vi "getFilePaths.vi"(8 "error in (no error)":errorcluster, 11 "reference in":refnum<class "File Controller.lvclass">) -> (0 "error out":errorcluster, 3 "reference out":refnum<class "File Controller.lvclass">)   [LabVIEW 2015, in "File Controller.lvclass"]
uses:
  File Controller.lvclass
  <vilib>/Utility/config.llb/Read Key (Path).vi
  <vilib>/Utility/config.llb/NI_LVConfig.lvlib
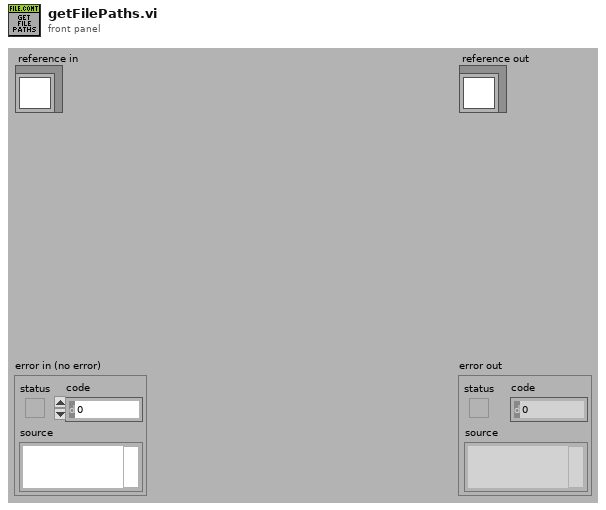
[diagram p1: front panel]
types:
  T1 = typedef "File Controller.lvclass/ObjectAttributesRef.ctl" = refnum<data-value>
  T2 = typedef "File Controller.lvclass/ObjectAttributes.ctl" = cluster{"MyAttribute":dbl, "excelFile_refs":refnum<class "excelFile.lvclass">[], "filePaths":path[], "outlookTemplatePaths":path[], "attachmentTemplatePaths":path[], "configFilePath":path, "not_setting":bool[], "python_ref":refnum<class "python.lvclass">, "TSR":cluster{"number":string, "TSR_path":path, "service_path":path, "email_to":string}}
  T3 = typedef "NI_LVConfig.lvlib/Config Data RefNum.ctl" = refnum<k1>
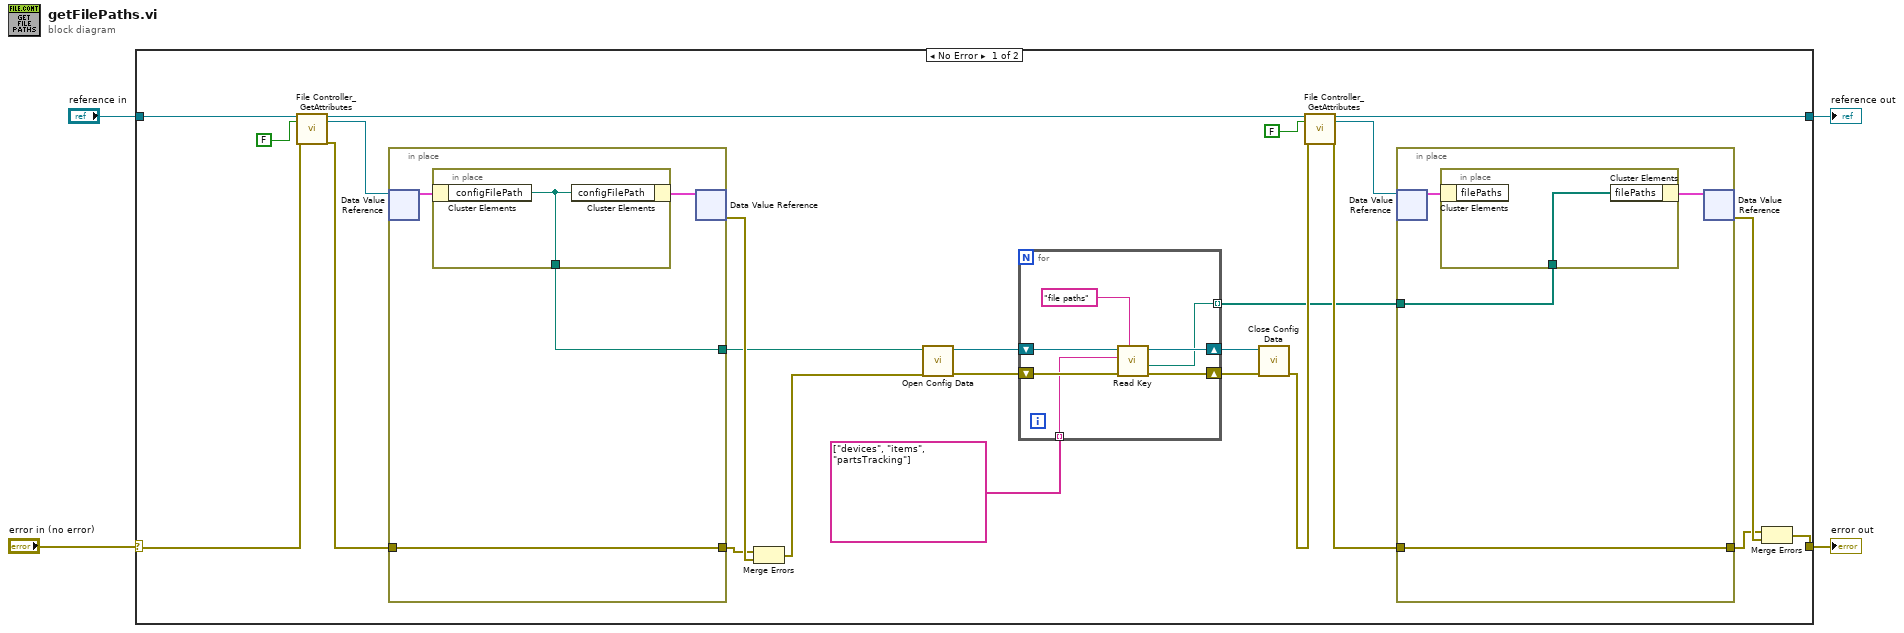
[diagram p0: block diagram]
diagram:
  n1 = case shown="No Error" "error in (no error)" {
    selector: "error in (no error)" -> [w9 w47]
    tunnel: [w28 w47] -> w3
    tunnel: [w23 w46] -> w1
    tunnel: "reference in" -> [w8 w46]
    frame No Error {
      n2 = call "File Controller_GetAttributes.vi"("reference in"=w8, "return data? (T)"=FALSE, "error in (no error)"=w9) -> ("reference out"=w7:refnum<class "File Controller.lvclass">, "attributes ref"=w10:T1, "error out"=w11:errorcluster)  [unwired: 13 in, 1 out]
      n3 = in-place {
        in-place-border: w11 -> [w30]
        in-place-border: [w30] -> w13
        in-place-border: [w29] -> w6
        n4 = in-place-dvr #1(w10) -> (w31:T2)  [unwired: 1 out]
        n5 = in-place {
          in-place-border: [w33] -> w29
          n6 = in-place-cluster #2(w31) -> ("configFilePath"=w33:path)
          n7 = in-place-cluster #2("configFilePath"=w33) -> (w32:T2)
        }
        n8 = in-place-dvr #1(w32) -> (w14:errorcluster)  [unwired: 1 out]
      }
      n9 = Merge Errors(w13, w14) -> (w5:errorcluster)
      n10 = call <vilib>:"Open Config Data.vi"("error in (no error)"=w5, "configuration file path"=w6) -> ("error out"=w20:errorcluster, "refnum"=w21:T3)  [unwired: 7 in, 1 out]
      n11 = for {
        shift-right: [w37] -> w19
        shift-left: w21 -> [w40]
        shift-right: [w36] -> w18
        shift-left: w20 -> [w39]
        tunnel: string[] ["devices", "items", "partsTracking"] -> [w35] mode=indexing
        tunnel: [w34] -> w15 mode=indexing
        n12 = call-poly <vilib>:"Read Key.vi"("section"="file paths", "error in (no error)"=w39, "key"=w35, "refnum"=w40) -> ("error out"=w36:errorcluster, "value"=w34:path, "refnum out"=w37:T3)  [unwired: 4 in, 1 out]
      }
      n13 = call <vilib>:"Close Config Data.vi"("error in (no error)"=w18, "refnum"=w19) -> ("error out"=w16:errorcluster)  [unwired: 8 in, 1 out]
      n14 = call "File Controller_GetAttributes.vi"("reference in"=w7, "return data? (T)"=FALSE, "error in (no error)"=w16) -> ("reference out"=w23:refnum<class "File Controller.lvclass">, "attributes ref"=w22:T1, "error out"=w24:errorcluster)  [unwired: 13 in, 1 out]
      n15 = in-place {
        in-place-border: w24 -> [w42]
        in-place-border: [w42] -> w26
        in-place-border: w15 -> [w41]
        n16 = in-place-dvr #3(w22) -> (w43:T2)  [unwired: 1 out]
        n17 = in-place {
          in-place-border: w41 -> [w45]
          n18 = in-place-cluster #4(w43) -> ()  [unwired: 1 out]
          n19 = in-place-cluster #4("filePaths"=w45) -> (w44:T2)
        }
        n20 = in-place-dvr #3(w44) -> (w27:errorcluster)  [unwired: 1 out]
      }
      n21 = Merge Errors(w26, w27) -> (w28:errorcluster)
    }
    frame Error {
    }
  }
  "error out" <- w3
  "reference out" <- w1
